vi "Make Header Array.vi"(8 "error in (no error)":errorcluster, 10 "priority":i32, 11 "Serializable Msg in":refnum<class "Serializable Msg.lvclass">) -> (0 "error out":errorcluster, 3 "Serializable Msg out":refnum<class "Serializable Msg.lvclass">)   [LabVIEW 2020, in "Serializer.lvlib" / "Serializable Message.lvlib" / "Serializable Msg.lvclass"]
uses:
  Serializable Msg.lvclass
  Serializable Msg.lvclass/Serializable Msg.ctl
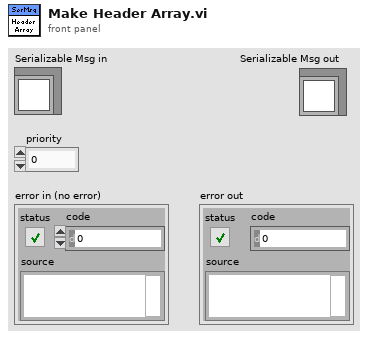
[diagram p1: front panel]
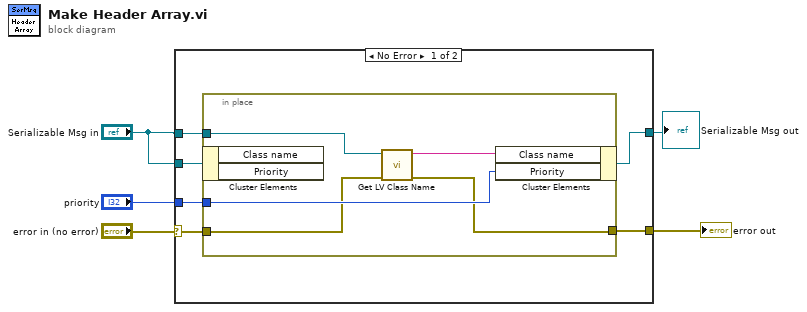
[diagram p0: block diagram]
diagram:
  n1 = case shown="No Error" "error in (no error)" {
    selector: "error in (no error)" -> [w9 w18]
    tunnel: "priority" -> [w11 _]
    tunnel: "Serializable Msg in" -> [w10 _]
    tunnel: [w8 w18] -> w3
    tunnel: "Serializable Msg in" -> [w7 w17]
    tunnel: [w6 w17] -> w1
    frame No Error {
      n2 = in-place "In Place Element Structure" {
        in-place-border: w11 -> [w16]
        in-place-border: w7 -> [w15]
        in-place-border: w9 -> [w13]
        in-place-border: [w12] -> w8
        n3 = in-place-cluster #1(w10) -> ()  [unwired: 2 out]
        n4 = call <vilib>:"Get LV Class Name.vi"("error in (no error)"=w13, "object"=w15) -> ("error out"=w12:errorcluster, "class name"=w14:string)  [unwired: 8 in]
        n5 = in-place-cluster #1("Class name"=w14, "Priority"=w16) -> (w6:refnum<class "Serializable Msg.lvclass">)
      }
    }
    frame Error {
    }
  }
  "error out" <- w3
  "Serializable Msg out" <- w1
